vi "ex01_g.vi"() -> ()   [LabVIEW 2011]
panel:
  out "Numeric Indicator 2":i64
  in  "Combo Box":string(combo)
  in  "stop":bool
  out "Boolean 3":bool
  in  "OK Button":bool
  in  "Boolean 2":bool
  out "Numeric Indicator":i64
  in  "Numeric Control":dbl
  out "Boolean":bool
  out "Gauge":dbl(knob) scale=0.1..100.0
  in  "Knob":dbl(knob) scale=0.0..100.0
  out "Numeric 2":dbl
  in  "Numeric":dbl
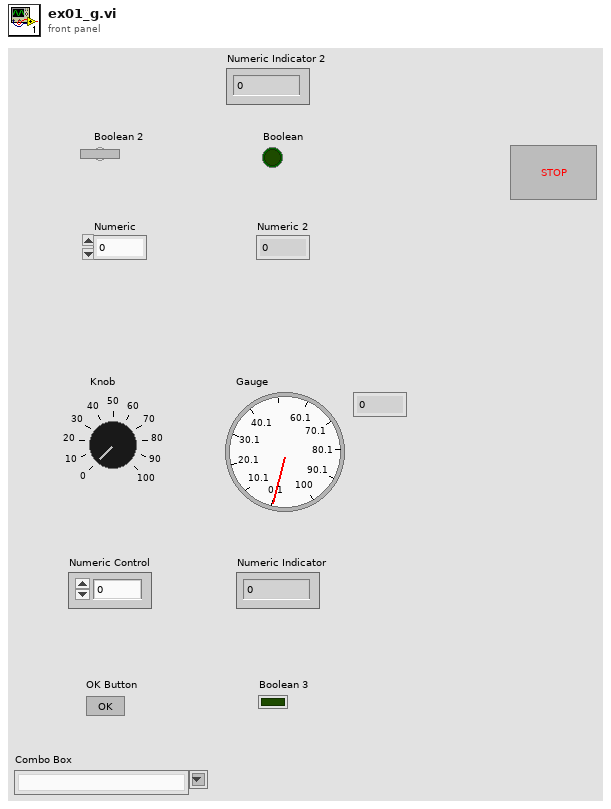
[diagram p1: front panel]
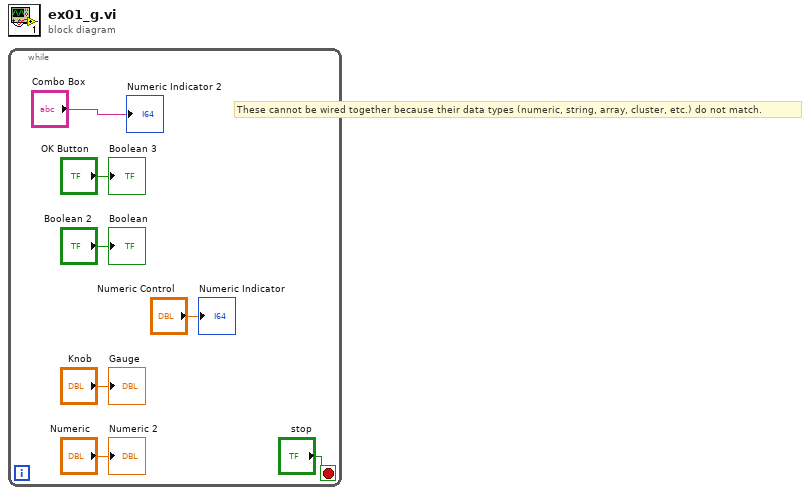
[diagram p0: block diagram]
diagram:
  # "These cannot be wired together because their data types (numeric, string, array, cluster, etc.) do not match."
  n1 = while {
    stop <- "stop" stop-if-true
    "Numeric 2" <- "Numeric"
    "Gauge" <- "Knob"
    "Boolean" <- "Boolean 2"
    "Numeric Indicator" <- "Numeric Control"
    "Boolean 3" <- "OK Button"
    "Numeric Indicator 2" <- "Combo Box"
  }
